vi "Check Frames Done.vi"(8 "Increment?":bool, 9 "Frames Finished":u32, 11 "Frames to Acquire":u32) -> (1 "Updated Frames Finished":u32, 2 "Is NumFrames >0?":bool, 3 "Frames Done?":bool)   [LabVIEW 2014]
panel:
  # "Copyright 2014 Vidrio Technologies\nScanImage 5 software is licensed under the Apache License, Version 2.0 (the \"License\"); you may not use any files contained\nwithin the ScanImage 5 release except in compliance with the License. You may obtain a copy of the License at\n http://www.apache.org/licenses/LICENSE-2.0\nUnless required by applicable law or agreed to in writing, software distributed under the License is distributed on an\n\"AS IS\" BASIS, WITHOUT WARRANTIES OR CONDITIONS OF ANY KIND, either express or implied. See the License for the\n specific language governing permissions and limitations under the License."
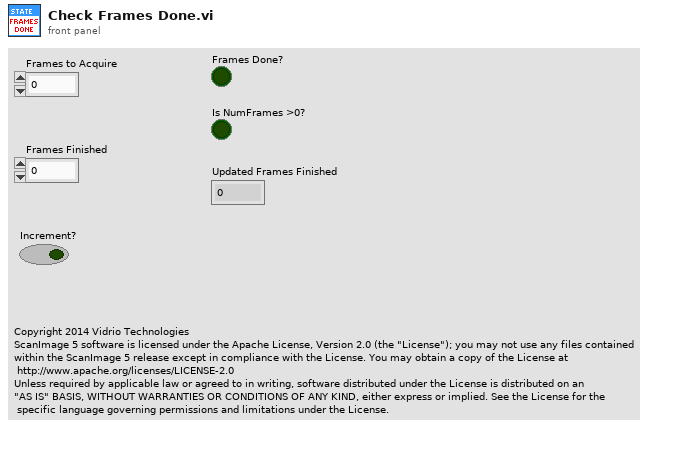
[diagram p1: front panel]
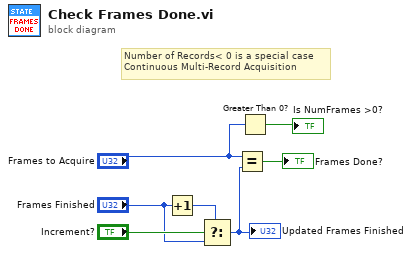
[diagram p0: block diagram]
diagram:
  # "Number of Records< 0 is a special case\nContinuous Multi-Record Acquisition"
  n1 = Increment(x="Frames Finished") -> (x+1=w7:u32)
  n2 = Select(t=w7, s="Increment?", f="Frames Finished") -> (s? t:f=w4:u32)
  "Updated Frames Finished" <- w4
  n3 = Equal?(x="Frames to Acquire", y=w4) -> (x = y?=→"Frames Done?":bool)
  n4 = Greater Than 0?(x="Frames to Acquire") -> (x > 0?=→"Is NumFrames >0?":bool)
